vi "opencvSegmentMultipleTest.vi"() -> ()   [LabVIEW 2017]
uses:
  opencvSegmentConvertCoordinates-multiFrames.vi
  opencvSelectCandidateNeurons5Planes.vi
  opencvSegment.vi
  opencvSegmentConvertCoordinates-singleFrame.vi
panel:
  out "NeuronN[total]":u16
  out "NeuronXY[frame]":u16[][](array[numeric])
  out "NeuronN[frame]":u16[](array[numeric])
  in  "frame 0":i32=24
  in  "N frames":i32=24
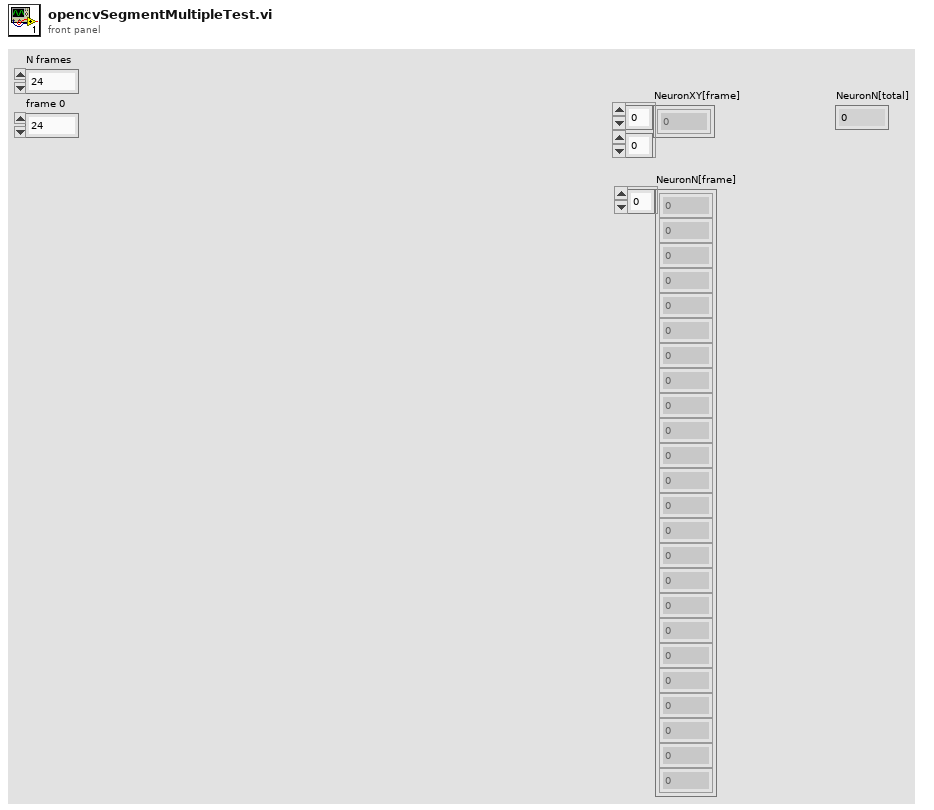
[diagram p1: front panel]
types:
  T1 = enum16{"big-endian, network order", "native, host order", "little-endian"}
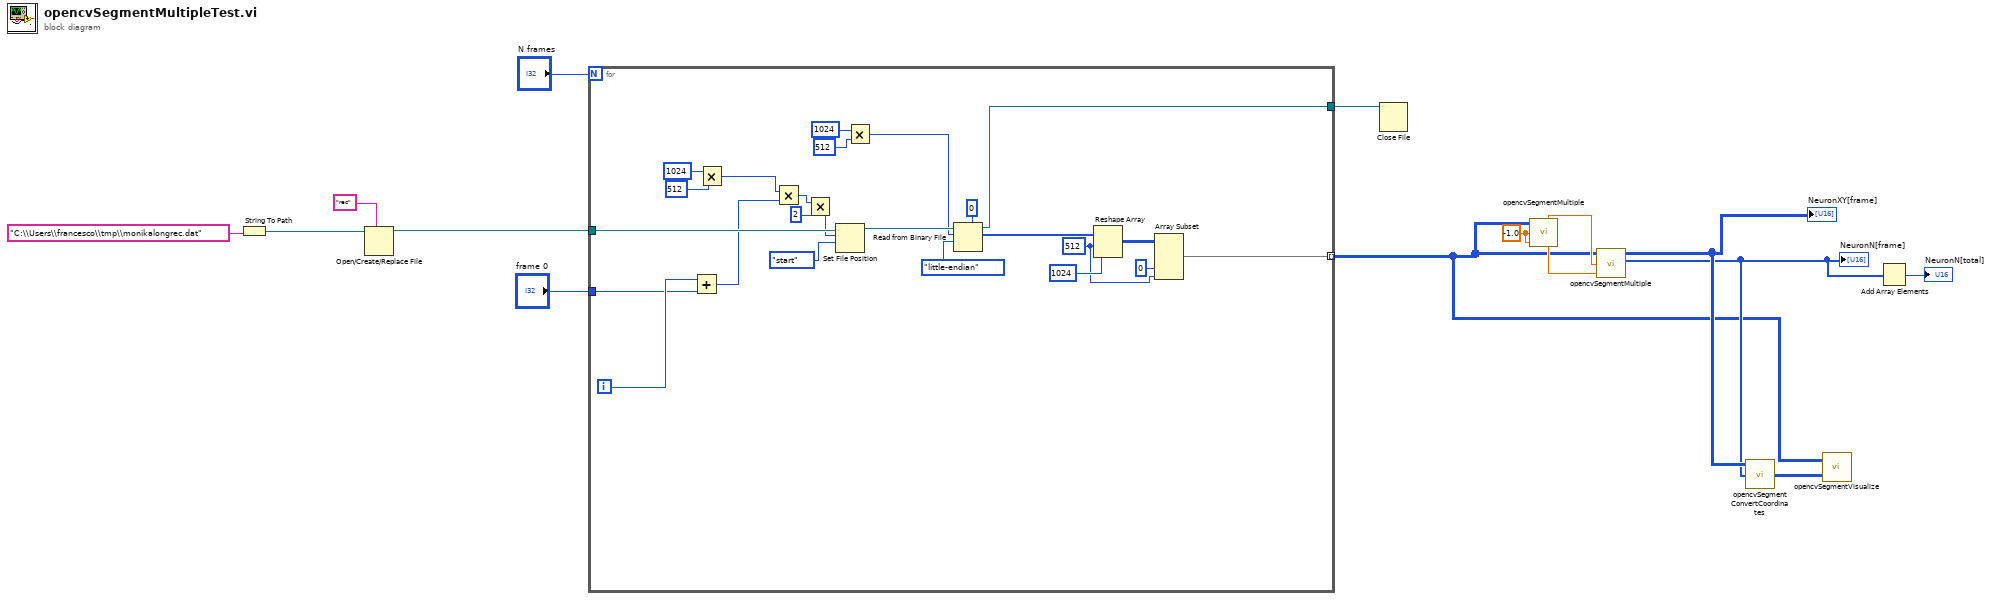
[diagram p0: block diagram]
diagram:
  w8 = -1.0 ("maxXInStack")
  n1 = String To Path(string="C:\\Users\\francesco\\tmp\\monikalongrec.dat") -> (path=w12:path)
  n2 = Open/Create/Replace File(file path (use dialog)=w12, prompt="rec") -> (refnum out=w15:refnum<file>)  [unwired: 4 in, 2 out]
  n3 = for {
    N: "N frames" -> [_]
    tunnel: w15 -> [w33]
    tunnel: [w22] -> w10
    tunnel: [w18] -> w1 mode=indexing
    tunnel: "frame 0" -> [w20]
    i -> [w21]
    w16 = 512 ("dimension size")
    n4 = Add(x=w21, y=w20) -> (x+y=w19:i32)
    n5 = Multiply(x=i64 1024, y=i64 512) -> (x*y=w32:i64)
    n6 = Multiply(x=w32, y=w19) -> (x*y=w29:i64)
    n7 = Multiply(x=w29, y=i64 2) -> (x*y=w27:i64)
    n8 = Set File Position(offset (in bytes) (0)=w27, refnum=w33, from (0:start)=enum16{"start", "end", "current"}."start") -> (refnum out=w31:refnum<file>)  [unwired: 1 in, 1 out]
    n9 = Multiply(x=1024, y=512) -> (x*y=w25:i32)
    n10 = Read from Binary File(5:u16 0, 9:T1."little-endian" ("byte order (0:big-endian, network order)"), 10:w25, 11:w31) -> (2:w34:u16[], 3:w22:refnum<file>)  [unwired: 2 in, 2 out]
    n11 = Reshape Array(w34, w16, 1024 ("dimension size")) -> (w23:u16[][])
    n12 = Array Subset(array=w23, index (col)=0 ("index"), length (col)=w16) -> (w18:u16[][])  [unwired: 2 in]
  }
  n13 = Close File(refnum=w10) -> ()  [unwired: 1 in, 2 out]
  n14 = call "opencvSegmentMultiple.vi"("maxYInStack"=w8, "maxXInStack"=w8, "ImgIn"=w1) -> ("maxY"=w7:dbl, "maxX"=w6:dbl)  [unwired: 4 out]
  n15 = call "opencvSegmentMultiple.vi"("maxYInStack"=w7, "maxXInStack"=w6, "ImgIn"=w1) -> ("NeuronN[frame]"=w3:u16[], "NeuronXY[frame]"=w4:u16[][])  [unwired: 4 out]
  "NeuronN[frame]" <- w3
  "NeuronXY[frame]" <- w4
  n16 = call-poly "opencvSegmentConvertCoordinates.vi"("NeuronN"=w3, "NeuronXY"=w4) -> ("XY"=w2:u16[][][])  [unwired: 1 in]
  n17 = call "opencvSegmentVisualize.vi"("XY"=w2, "ImgIn"=w1) -> ()  [unwired: 1 in]
  n18 = Add Array Elements(numeric array=w3) -> (sum=→"NeuronN[total]":u16)
